vi "PH_PP_CurrentMeas.PC Write PSDB.vi"(0 "i ref in":refnum<vi>, 5 "error IO":errorcluster) -> (14 "i ref out":refnum<vi>, 19 "error out":errorcluster)   [LabVIEW 2014, in "PH_PP_CurrentMeas.lvlib"]
doc: "This is the proc case which writes data to the PHELIX shot data base."
uses:
  PH_PP_CurrentMeas.lvlib
  User/Eisenbarth/psdb_lv/PSDB_AxisDescription.ctl
  PH_PSDBWriter/PH_PSDBWriter.2D dataset.ctl
  PH_Common/PH_Common.lvlib
  User/Eisenbarth/psdb_lv/PSDB.lvlib
  PH_PSDBWriter/PH_PSDBWriter.lvlib
  PH_StatusHandler/PH_StatusHandler.lvlib
panel:
  in  "2D data":T1
  in  "axis description":T2
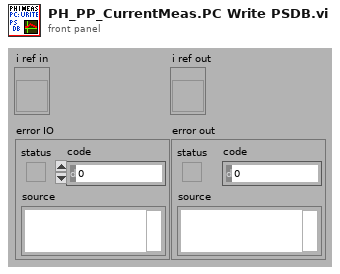
[diagram p1: front panel]
types:
  T1 = typedef "PH_PSDBWriter.lvlib/PH_PSDBWriter.2D dataset.ctl" = cluster{"name":string, "data":dbl[][], "axis description":T2}
  T2 = typedef "PSDB.lvlib/PSDB_AxisDescription.ctl" = cluster{"x axis label":string, "y axis label":string, "x axis unit":string, "y axis unit":string}
  T3 = typedef "PH_PP_CurrentMeas.lvlib/PH_PP_CurrentMeas.i attribute.ctl" = cluster{"Status":cluster{"GUI Ref Hardware Feedback":refnum<vi>, "Tab Control":refnum<vi>}, "PU 1":cluster{"Instance":string, "Status":T4, "Ref Status ":refnum<vi>, "Data":waveform(dbl)[], "Ref Data":refnum<vi>}, "PU 2":cluster{"Instance":string, "Status":T4, "Ref Status ":refnum<vi>, "Data":waveform(dbl)[], "Ref Data":refnum<vi>}, "PU 3":cluster{"Instance":string, "Status":T4, "Ref Status ":refnum<vi>, "Data":waveform(dbl)[], "Ref Data":refnum<vi>}, "PU 4":cluster{"Instance":string, "Status":T4, "Ref Status ":refnum<vi>, "Data":waveform(dbl)[], "Ref Data":refnum<vi>}, "PU 5":cluster{"Instance":string, "Status":T4, "Ref Status ":refnum<vi>, "Data":waveform(dbl)[], "Ref Data":refnum<vi>}, "FR":cluster{"Instance":string, "Status":T4, "Ref Status ":refnum<vi>, "Data":waveform(dbl)[], "Ref Data":refnum<vi>}, "PA - 19mm 1":cluster{"Instance":string, "Status":T4, "Ref Status ":refnum<vi>}, "PA - 19mm 2":cluster{"Instance":string, "Status":T4, "Ref Status ":refnum<vi>, "no link":bool}, "PA - 45mm":cluster{"Instance":string, "Status":T4, "Ref Status ":refnum<vi>, "no link":bool}, "PA Data":cluster{"Data":waveform(dbl)[], "Ref":refnum<vi>}, "Sequencer":cluster{"Instance":string, "SM State Ref":refnum<vi>}, "Tasks":cluster{"Port":u16, "connection ID":refnum<k5>, "Status":T4, "Ref":refnum<vi>, "Ref Bar":refnum<vi>, "Feedback":cluster{"Received Data Sets":T5[], "Driver Error":errorcluster, "Connection not established":bool, "Error unpacking the data":bool, "No Task defined":bool, "Not triggered yet":bool}, "Data":waveform(dbl)[], "Ref Teststart Task":refnum<vi>}[], "in use":cluster{"MA DP":bool, "FR and PA":bool}, "DAQ Server":string}
  T4 = typedef "PH_StatusHandler.lvlib/PH_StatusHandler.Status.ctl" = i16
  T5 = typedef "PH_PP_CurrentMeas.lvlib/PH_PP_CurrentMeas.CommandCluster.ctl" = cluster{"Command":string, "Data":string, "error out":errorcluster}
  T6 = cluster{"Port":u16, "connection ID":refnum<k5>, "Status":T4, "Ref":refnum<vi>, "Ref Bar":refnum<vi>, "Feedback":cluster{"Received Data Sets":T5[], "Driver Error":errorcluster, "Connection not established":bool, "Error unpacking the data":bool, "No Task defined":bool, "Not triggered yet":bool}, "Data":waveform(dbl)[], "Ref Teststart Task":refnum<vi>}[]
  T7 = typedef "PH_PSDBWriter.lvlib/PH_PSDBWriter.Numeric dataset.ctl" = cluster{"name":string, "data":dbl, "unit":string}
  T8 = typedef "PH_PSDBWriter.lvlib/PH_PSDBWriter.String dataset.ctl" = cluster{"name":string, "data":string, "unit":string}
  T9 = typedef "PH_PSDBWriter.lvlib/PH_PSDBWriter.PSDB Dataset.ctl" = cluster{"Version":i32, "2D data Input":T1[], "Boolean Input":T10[], "Image Input":T11[], "Numeric Input":T7[], "String Input":T8[]}
  T10 = typedef "PH_PSDBWriter.lvlib/PH_PSDBWriter.Boolean dataset.ctl" = cluster{"name":string, "data":bool, "unit":string}
  T11 = typedef "PH_PSDBWriter.lvlib/PH_PSDBWriter.Image dataset.ctl" = cluster{"name":string, "data":T12, "unit":string}
  T12 = typedef "IMAQ Image.ctl" = refnum<image>
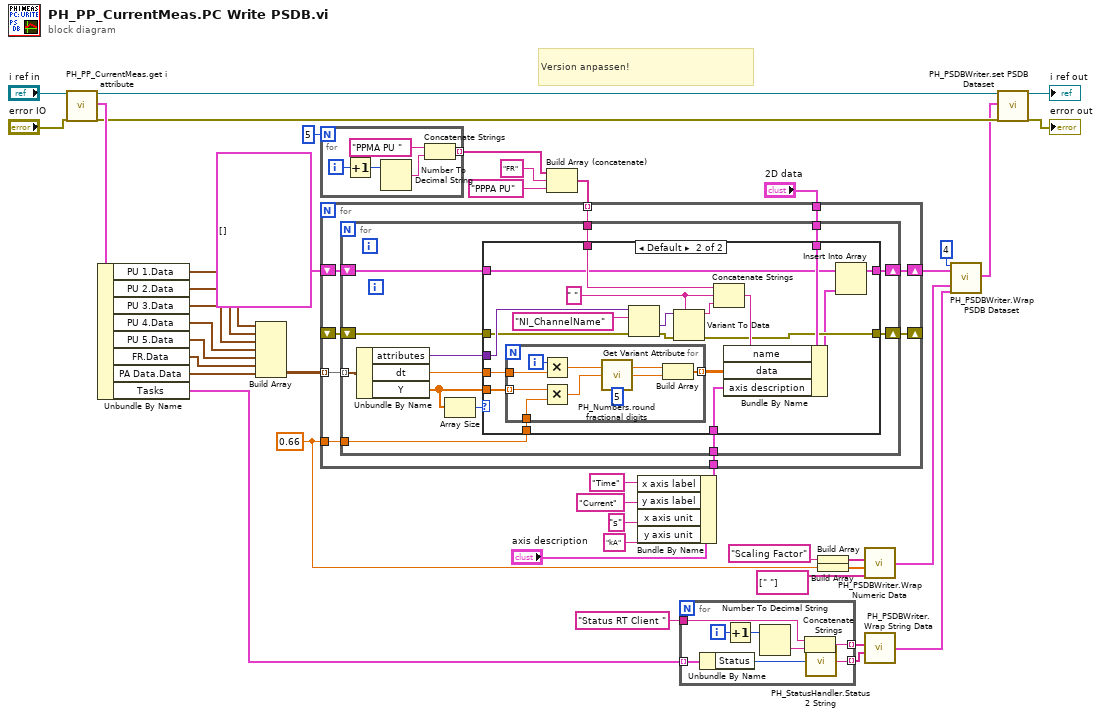
[diagram p0: block diagram]
diagram:
  w8 = 0.66 ("data")
  # "Version anpassen!"
  n1 = call "PH_PP_CurrentMeas.get i attribute.vi"("i ref in"="i ref in", "error in (no error)"="error IO") -> ("i ref out"=w16:refnum<vi>, "i attribute"=w21:T3, "error out"=w20:errorcluster)  [unwired: 15 in]
  n2 = Unbundle By Name(w21) -> ("PU 1.Data"=w40:waveform(dbl)[], "PU 2.Data"=w39:waveform(dbl)[], "PU 3.Data"=w37:waveform(dbl)[], "PU 4.Data"=w36:waveform(dbl)[], "PU 5.Data"=w35:waveform(dbl)[], "FR.Data"=w34:waveform(dbl)[], "PA Data.Data"=w33:waveform(dbl)[], "Tasks"=w5:T6)
  n3 = Build Array(w40, w39, w37, w36, w35, w34, w33) -> (w38:waveform(dbl)[][])
  n4 = for {
    N: 5 -> [_]
    tunnel: [w43] -> w30 mode=indexing
    i -> [w47]
    n5 = Increment(x=w47) -> (x+1=w46:i32)
    n6 = Number To Decimal String(number=w46) -> (decimal integer string=w44:string)  [unwired: 1 in]
    n7 = Concatenate Strings("PPMA PU ", w44) -> (w43:string)
  }
  n8 = Build Array (concatenate)(w30, "FR", "PPPA PU") -> (w11:string[])
  n9 = Bundle By Name(cluster="axis description", "x axis label"="Time", "y axis label"="Current", "x axis unit"="s", "y axis unit"="kA") -> (w27:T2)
  n10 = for {
    tunnel: w38 -> [w56] mode=indexing
    tunnel: w8 -> [w55]
    tunnel: w11 -> [w54] mode=indexing
    tunnel: w27 -> [w53]
    shift-right: [w52] -> _
    shift-left: _ -> [w51]
    tunnel: "2D data" -> [w50]
    shift-right: [w49] -> w12
    shift-left: T1[] [] -> [w48]
    n11 = for {
      tunnel: w56 -> [w69] mode=indexing
      tunnel: w55 -> [w68]
      tunnel: w54 -> [w65]
      shift-right: [w64] -> w52
      shift-left: w51 -> [w63]
      tunnel: w53 -> [w62]
      tunnel: w50 -> [w59]
      shift-right: [w58] -> w49
      shift-left: w48 -> [w57]
      n12 = Unbundle By Name(w69) -> ("attributes"=w67:variant, "dt"=w66:dbl, "Y"=w61:dbl[])
      n13 = Array Size(array=w61) -> (size(s)=w60:i32)
      n14 = case shown="Default" w60 {
        tunnel: w68 -> [_ w90]
        tunnel: w67 -> [_ w89]
        tunnel: w66 -> [_ w86]
        tunnel: w65 -> [_ w83]
        tunnel: [w71 w75] -> w64
        tunnel: w63 -> [w71 w81]
        tunnel: w62 -> [_ w76]
        tunnel: w61 -> [_ w80]
        tunnel: w59 -> [_ w79]
        tunnel: [w70 w73] -> w58
        tunnel: w57 -> [w70 w72]
        frame 0 {
        }
        frame Default {
          w82 = " " ("string")
          n15 = for {
            tunnel: w86 -> [w97]
            tunnel: w80 -> [w99] mode=indexing
            tunnel: w90 -> [w98]
            tunnel: [w94] -> w77 mode=indexing
            i -> [w96]
            n16 = Multiply(x=w96, y=w97) -> (x*y=w95:dbl)
            n17 = Multiply(x=w99, y=w98) -> (x*y=w93:dbl)
            n18 = call "PH_Numbers.round fractional digits.vi"("Input"=w93, "Position (1)"=i16 5) -> ("round Output"=w92:dbl)
            n19 = Build Array(w95, w92) -> (w94:dbl[])
          }
          n20 = Get Variant Attribute(Variant=w89, name="NI_ChannelName", error in=w81) -> (value=w87:variant, error out=w88:errorcluster)  [unwired: 1 in, 2 out]
          n21 = Variant To Data(error in=w88, type=w82, Variant=w87) -> (data=w84:string, error out=w75:errorcluster)
          n22 = Concatenate Strings(w83, w82, w84) -> (w78:string)
          n23 = Bundle By Name(cluster=w79, "name"=w78, "data"=w77, "axis description"=w76) -> (w74:T1)
          n24 = Insert Into Array(array=w72, new element=w74) -> (w73:T1[])  [unwired: 1 in]
        }
      }
    }
  }
  n25 = for {
    tunnel: "Status RT Client " ("string") -> [w104]
    tunnel: w5 -> [w103] mode=indexing
    tunnel: [w101] -> w2 mode=indexing
    tunnel: [w100] -> w3 mode=indexing
    i -> [w107]
    n26 = Unbundle By Name(w103) -> ("Status"=w102:T4)
    n27 = Increment(x=w107) -> (x+1=w106:i32)
    n28 = Number To Decimal String(number=w106) -> (decimal integer string=w105:string)  [unwired: 1 in]
    n29 = Concatenate Strings(w104, w105) -> (w100:string)
    n30 = call "PH_StatusHandler.Status 2 String.vi"("Status"=w102) -> ("Status as string"=w101:string)
  }
  n31 = Build Array("Scaling Factor" ("name")) -> (w6:string[])
  n32 = Build Array(w8) -> (w7:dbl[])
  n33 = call "PH_PSDBWriter.Wrap Numeric Data.vi"("Unit Array"=string[] [" "], "Data Array"=w7, "Name Array"=w6) -> ("PSDB Numeric Data Array"=w10:T7[])  [unwired: 1 in]
  n34 = call "PH_PSDBWriter.Wrap String Data.vi"("Data Array"=w2, "Name Array"=w3) -> ("PSDB String Data Array"=w4:T8[])  [unwired: 2 in]
  n35 = call "PH_PSDBWriter.Wrap PSDB Dataset.vi"("Version"=4, "2D data Input"=w12, "Numeric Input"=w10, "String Input"=w4) -> ("PSDB Dataset"=w14:T9)  [unwired: 15 in]
  n36 = call "PH_PSDBWriter.set PSDB Dataset.vi"("VI in"=w16, "PSDB Dataset"=w14, "error in (no error)"=w20) -> ("VI out"=→"i ref out":refnum<vi>, "error out"=→"error out":errorcluster)  [unwired: 15 in]
